vi "IsEventEqual.vi"(8 "error in (no error)":errorcluster, 10 "EventToken":refnum<class "EventToken.lvclass">, 11 "EventToken in":refnum<class "EventToken.lvclass">) -> (0 "error out":errorcluster, 1 "Is Event Equal?":bool, 2 "EventToken":refnum<class "EventToken.lvclass">, 3 "EventToken out":refnum<class "EventToken.lvclass">)   [LabVIEW 2021, in "EventManagerLibrary.lvlib" / "EventToken.lvclass"]
doc: "Returns TRUE if two tokens refer to the same event."
uses:
  EventToken.lvclass
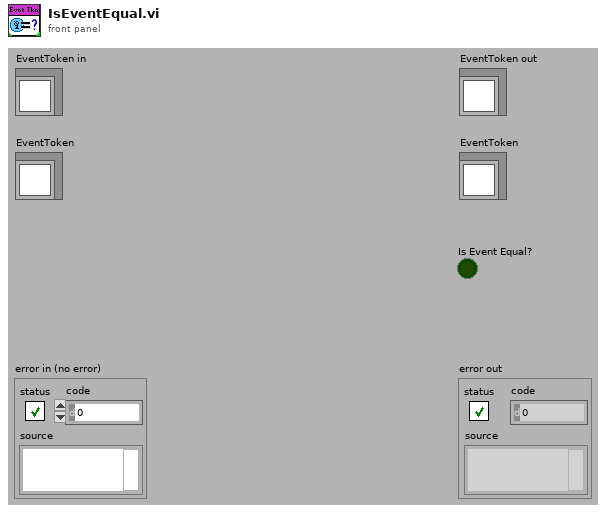
[diagram p1: front panel]
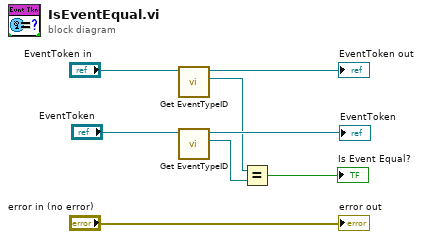
[diagram p0: block diagram]
diagram:
  n1 = call "Get EventTypeID.vi"("EventToken in"="EventToken in") -> ("EventData Class"=w2:refnum<class "EventData.lvclass">, "EventToken out"=→"EventToken out":refnum<class "EventToken.lvclass">)  [unwired: 8 in, 1 out]
  n2 = call "Get EventTypeID.vi"("EventToken in"="EventToken") -> ("EventData Class"=w1:refnum<class "EventData.lvclass">, "EventToken out"=→"EventToken":refnum<class "EventToken.lvclass">)  [unwired: 8 in, 1 out]
  n3 = Equal?(x=w2, y=w1) -> (x = y?=→"Is Event Equal?":bool)
  "error out" <- "error in (no error)"
